vi "SweepStepArray_DP_Ver1.0.vi"(2 "CMD Head&Format":string, 4 "# of total points:":u32=100 step=1, 5 "# of sweep steps:":u32=100 step=1, 6 "Manual Array":sgl[](array[numeric]) format="%.2f", 7 "Sweep Mode":u8(ring) items=["Linear", "Log", "Exp", "Inverse", "Manual"], 8 "Stop":dbl, 9 "Start":dbl) -> (0 "Array Out":dbl[](array[numeric]) format="%.4f", 1 "Stay duration points":dbl, 3 "VariableCMD Array out":string[](array[string]))   [LabVIEW 2011]
doc: "Ramp Type:\n0: Linear\n1: Log\n2: Exp\n3: Inverse\n4: Output Input Array\n>5 : Linear\nWatch out the input value is valid or not"
uses:
  <vilib>/Analysis/1siggen.llb/Ramp Pattern by Samples.vi
  <vilib>/Analysis/NI_AALBase.lvlib
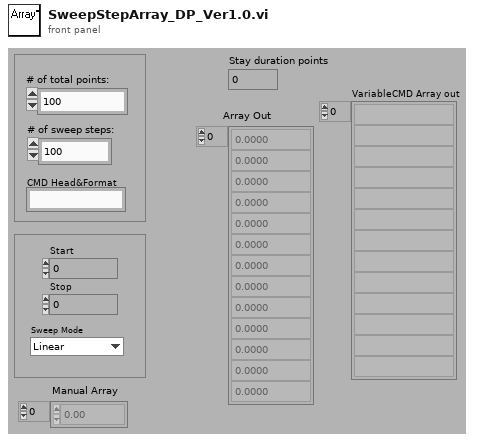
[diagram p1: front panel]
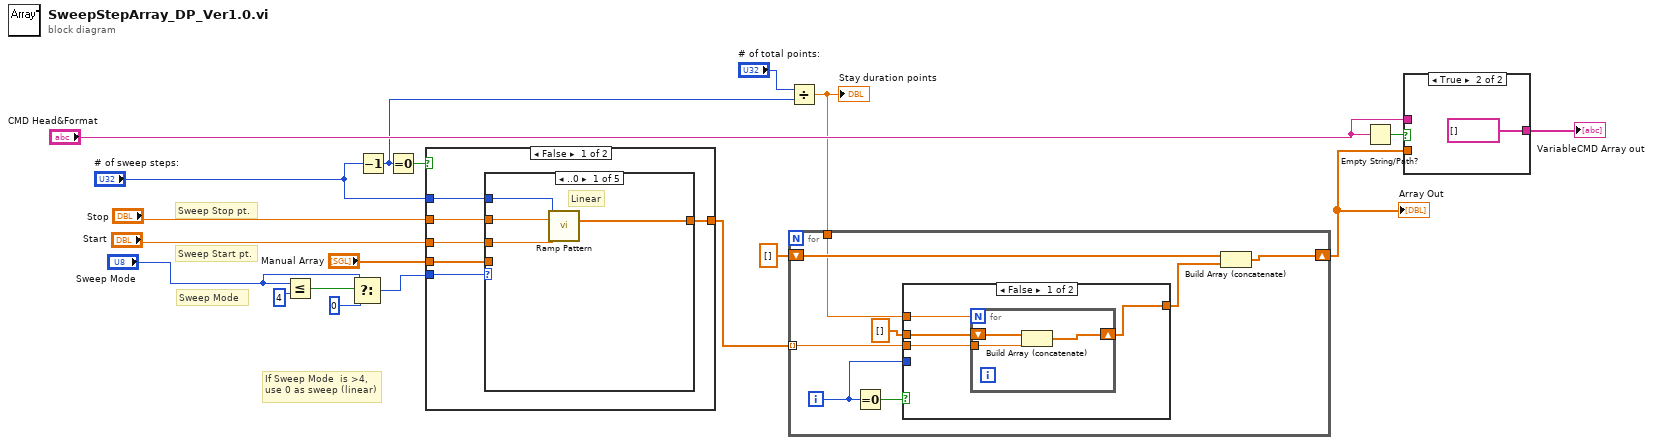
[diagram p0: block diagram]
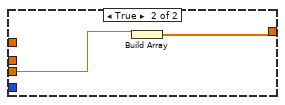
[diagram p2: hidden frame]
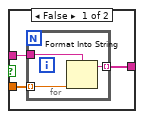
[diagram p3: hidden frame]
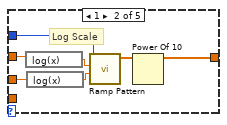
[diagram p4: hidden frame]
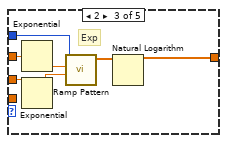
[diagram p5: hidden frame]
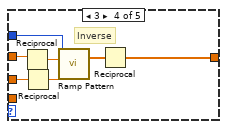
[diagram p6: hidden frame]
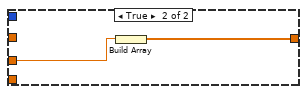
[diagram p8: hidden frame]
diagram:
  # "Sweep Mode"
  # "Sweep Start pt."
  # "Sweep Stop pt."
  # "If Sweep Mode  is >4,\nuse 0 as sweep (linear)"
  n1 = Less Or Equal?(x="Sweep Mode", y=u8 4) -> (x <= y?=w14:bool)
  n2 = Select(t="Sweep Mode", s=w14, f=u8 0) -> (s? t:f=w17:u8)
  n3 = Decrement(x="# of sweep steps:") -> (x-1=w1:u32)
  n4 = Equal To 0?(x=w1) -> (x = 0?=w18:bool)
  n5 = case shown="False" w18 {
    tunnel: "# of sweep steps:" -> [w25 _]
    tunnel: [w24 w52] -> w4
    tunnel: "Start" -> [w23 w53]
    tunnel: "Stop" -> [w22 _]
    tunnel: "Manual Array" -> [w21 _]
    tunnel: w17 -> [w20 _]
    frame False {
      n6 = case shown="..0" w20 {
        tunnel: [w27 w36 w43 w46 w51] -> w24
        tunnel: w21 -> [_ _ _ _ w51]
        tunnel: w25 -> [w29 w35 w40 w50 _]
        tunnel: w22 -> [w26 w33 w42 w47 _]
        tunnel: w23 -> [w28 w30 w41 w49 _]
        frame ..0 {
          # "Linear"
          n7 = call-poly <vilib>:"Ramp Pattern.vi"("start"=w28, "end"=w26, "samples"=w29) -> ("Ramp Pattern"=w27:dbl[])  [unwired: 7 in, 1 out]
        }
        frame 1 {
          # "Log Scale"
          n8 = expression code="log(x)"(w33) -> (w32:dbl)
          n9 = expression code="log(x)"(w30) -> (w31:dbl)
          n10 = call-poly <vilib>:"Ramp Pattern.vi"("start"=w31, "end"=w32, "samples"=w35) -> ("Ramp Pattern"=w34:dbl[])  [unwired: 7 in, 1 out]
          n11 = Power Of 10(x=w34) -> (10^x=w36:dbl[])
        }
        frame 2 {
          # "Exp"
          n12 = Exponential(1:w42) -> (0:w39:dbl)
          n13 = Exponential(1:w41) -> (0:w38:dbl)
          n14 = call-poly <vilib>:"Ramp Pattern.vi"("start"=w38, "end"=w39, "samples"=w40) -> ("Ramp Pattern"=w37:dbl[])  [unwired: 7 in, 1 out]
          n15 = Natural Logarithm(1:w37) -> (0:w43:dbl[])
        }
        frame 3 {
          # "Inverse"
          n16 = Reciprocal(x=w47) -> (1/x=w45:dbl)
          n17 = Reciprocal(x=w49) -> (1/x=w44:dbl)
          n18 = call-poly <vilib>:"Ramp Pattern.vi"("start"=w44, "end"=w45, "samples"=w50) -> ("Ramp Pattern"=w48:dbl[])  [unwired: 7 in, 1 out]
          n19 = Reciprocal(x=w48) -> (1/x=w46:dbl[])
        }
        frame 4.. {
          # "Manual"
        }
      }
    }
    frame True {
      n20 = Build Array(w53) -> (w52:dbl[])
    }
  }
  n21 = Divide(x="# of total points:", y=w1) -> (x/y=w3:dbl)
  "Stay duration points" <- w3
  n22 = for {
    tunnel: w4 -> [w57] mode=indexing
    tunnel: w3 -> [w56]
    shift-right: [w54] -> w2
    shift-left: dbl[] [] ("Ramp Pattern") -> [w60]
    i -> [w58]
    n23 = Equal To 0?(x=w58) -> (x = 0?=w61:bool)
    n24 = case shown="False" w61 {
      tunnel: [w63 w70] -> w59
      tunnel: w58 -> [_ _]
      tunnel: w57 -> [w62 w69]
      tunnel: w56 -> [w65 _]
      tunnel: dbl[] [] ("Ramp Pattern") -> [w64 _]
      frame False {
        n25 = for {
          N: w65 -> [_]
          tunnel: w62 -> [w67]
          shift-right: [w66] -> w63
          shift-left: w64 -> [w68]
          n26 = Build Array (concatenate)(w68, w67) -> (w66:dbl[])
        }
      }
      frame True {
        n27 = Build Array(w69) -> (w70:dbl[])
      }
    }
    n28 = Build Array (concatenate)(w60, w59) -> (w54:dbl[])
  }
  "Array Out" <- w2
  n29 = Empty String/Path?(string/path="CMD Head&Format") -> (empty?=w10:bool)
  n30 = case shown="True" w10 {
    tunnel: "CMD Head&Format" -> [w73 _]
    tunnel: w2 -> [w72 _]
    tunnel: [w71 string[] []] -> w8
    frame False {
      n31 = for {
        tunnel: w72 -> [w76] mode=indexing
        tunnel: [w75] -> w71 mode=indexing
        tunnel: w73 -> [w74]
        n32 = Format Into String(format string=w74, w76) -> (resulting string=w75:string)  [unwired: 2 in, 1 out]
      }
    }
    frame True {
    }
  }
  "VariableCMD Array out" <- w8
